vi "_UpdateTargetResFile.vi"(8 "error in (no error)":errorcluster, 10 "Polarity":enum32{"Positive", "Negative"}(radio), 11 "Path":path=path "C:/Users/Public/Molana/Instrument/Configuration/Current setting/Calibration/targetResolution.res") -> (0 "error out":errorcluster)   [LabVIEW 2015]
uses:
  Type/_Log Command.ctl
  Type/_RT Command.ctl
  Configuration/_Global Configuration.vi
  <vilib>/xml/Load XML File.vi
  <vilib>/xml/Close Reference(Node).vi
  <vilib>/xml/NI_XML.lvlib
  <resource>/objmgr/DOMUserDefRef.rc
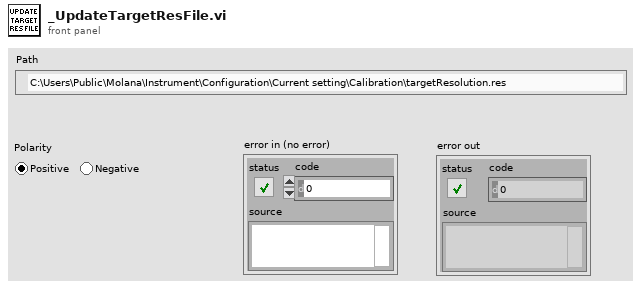
[diagram p1: front panel]
types:
  T1 = typedef "_Log Command.ctl" = enum16{"No Command", "Open", "Read", "Write", "Close", "Check Size"}
  T2 = typedef "_RT Command.ctl" = enum16{"xml Start Run", "xml Start Actual Run", "xml Stop Run", "xml Runtime Update", "xml Get Status", "xml Get Table", "xml Set Table", "xml Get Configuration", "xml System Status", "xml Set LC Input Logic", "xml Get Data", "xml Get Info", "Start", "StartActualRun", "Stop", "Runtime Update", "Get Data", "Get Info", "Get Status", "Get Param", "Get Config", "Get Table", "Read ADC", "Set Oscillator", "Update Config", "Update Table", "Set All Pol", "Set Pol and DC", "Set Max Mass", "Toggle RP", "Toggle EL", "Set PIC", "Initialize Turbo", "Send Turbo Comm", "Close Turbo", "P1", "P2", "P3", "Send Serial", "Set LC Out", "Get LC In", "Read VAC", "Test Table", "Toggle Power", "Get Startup", "Set Startup", "Get ADC Table", "Set ADC Table", "Get Brief Status", "Get Detail Status", "Auxiliary Update", "Set CC Logics", "Set CC Input Logics", "Ignore Error", "invalid"}
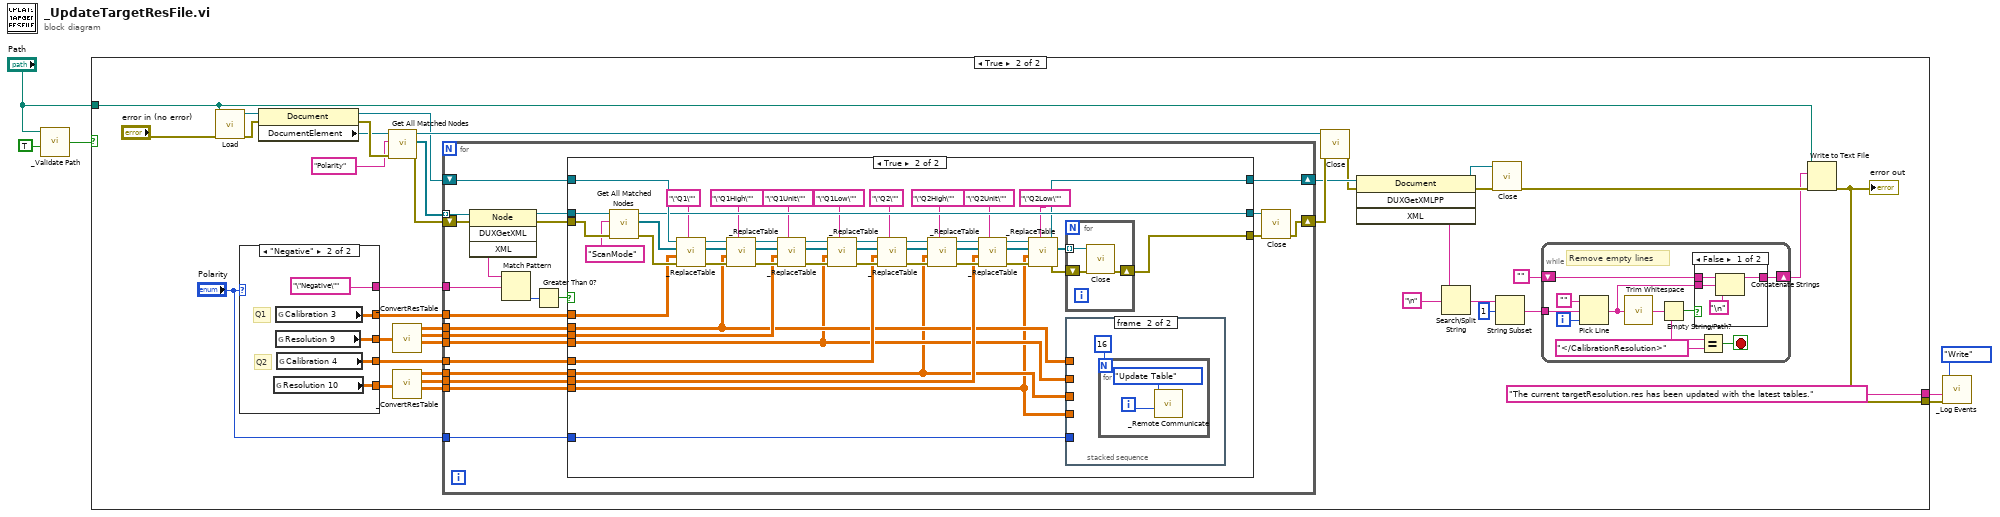
[diagram p0: block diagram]
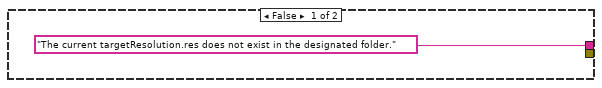
[diagram p2: hidden frame]
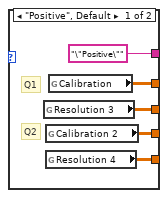
[diagram p4: hidden frame]
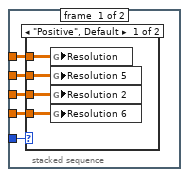
[diagram p6: hidden frame]
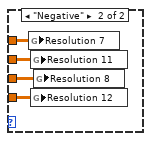
[diagram p7: hidden frame]
diagram:
  n1 = call "_Validate Path.vi"("Check Exist (F)"=TRUE, "path"="Path") -> ("Valid"=w4:bool)  [unwired: 2 in]
  n2 = case shown="True" w4 {
    tunnel: "Path" -> [_ w11]
    tunnel: ["The current targetResolution.res does not exist in the designated folder." ("initial string") "The current targetResolution.res has been updated with the latest tables." ("initial string")] -> w2
    tunnel: [_ w9] -> w1
    frame False {
    }
    frame True {
      n3 = call-poly <vilib>:"Load.vi"("path to XML document"=w11, "error in (no error)"="error in (no error)") -> ("DOM document out"=w45:refnum<k20>, "error out"=w44:errorcluster)  [unwired: 11 in, 1 out]
      n4 = case shown="\"Negative\"" "Polarity" {
        tunnel: ["\"Positive\"" "\"Negative\""] -> w38
        tunnel: [w64 w69] -> w32
        tunnel: [w63 w68] -> w34
        tunnel: [w62 w67] -> w31
        tunnel: [w61 w66] -> w33
        frame "Positive", Default {
          # "Q2"
          # "Q1"
          n5 = global read "_Global Configuration.vi" "Resolution 3"() -> (w63:dbl[][])
          n6 = global read "_Global Configuration.vi" "Calibration 2"() -> (w62:dbl[][])
          n7 = global read "_Global Configuration.vi" "Resolution 4"() -> (w61:dbl[][])
          n8 = global read "_Global Configuration.vi" "Calibration"() -> (w64:dbl[][])
        }
        frame "Negative" {
          # "Q2"
          # "Q1"
          n9 = global read "_Global Configuration.vi" "Resolution 10"() -> (w66:dbl[][])
          n10 = global read "_Global Configuration.vi" "Calibration 3"() -> (w69:dbl[][])
          n11 = global read "_Global Configuration.vi" "Resolution 9"() -> (w68:dbl[][])
          n12 = global read "_Global Configuration.vi" "Calibration 4"() -> (w67:dbl[][])
        }
      }
      n13 = property on="Property Node" class="Document"(reference=w45, error in=w44) -> (reference out=w35:refnum<k20>, error out=w43:errorcluster, "DocumentElement"=w42:refnum<k20>)
      n14 = call <vilib>:"Get All Matched Nodes.vi"("error in (no error)"=w43, "XPath expression"="Polarity", "node in"=w42) -> ("error out"=w40:errorcluster, "node result array"=w39:refnum<k20>[], "node out"=w36:refnum<k20>)  [unwired: 6 in]
      n15 = call "_ConvertResTable.vi"("ResTable"=w34) -> ("HiResTable"=w30:dbl[][], "MidResTable"=w29:dbl[][], "LowResTable"=w28:dbl[][])  [unwired: 1 in]
      n16 = call "_ConvertResTable.vi"("ResTable"=w33) -> ("HiResTable"=w27:dbl[][], "MidResTable"=w26:dbl[][], "LowResTable"=w25:dbl[][])  [unwired: 1 in]
      n17 = for {
        tunnel: w39 -> [w91] mode=indexing
        tunnel: w38 -> [w88]
        shift-right: [w86] -> w37
        shift-left: w40 -> [w92]
        shift-right: [w80] -> w24
        shift-left: w35 -> [w82]
        tunnel: w32 -> [w79]
        tunnel: w31 -> [w75]
        tunnel: w30 -> [w78]
        tunnel: w29 -> [w77]
        tunnel: w28 -> [w76]
        tunnel: w27 -> [w74]
        tunnel: w26 -> [w73]
        tunnel: w25 -> [w72]
        tunnel: "Polarity" -> [w71]
        n18 = invoke class="Node" method="DUXGetXML"(reference=w91, error in=w92) -> (reference out=w83:refnum<k20>, error out=w85:errorcluster, "XML"=w89:string)  [unwired: 2 in, 1 out]
        n19 = Match Pattern(string=w89, regular expression=w88) -> (offset past match=w90:i32)  [unwired: 1 in, 3 out]
        n20 = Greater Than 0?(x=w90) -> (x > 0?=w87:bool)
        n21 = case shown="True" w87 {
          tunnel: w85 -> [w95 w143]
          tunnel: [w95 w101] -> w84
          tunnel: w83 -> [w94 w144]
          tunnel: [w94 w139] -> w81
          tunnel: w82 -> [w93 w140]
          tunnel: [w93 w121] -> w80
          tunnel: w79 -> [_ w138]
          tunnel: w78 -> [_ w99]
          tunnel: w77 -> [_ w113]
          tunnel: w76 -> [_ w98]
          tunnel: w75 -> [_ w112]
          tunnel: w74 -> [_ w97]
          tunnel: w73 -> [_ w111]
          tunnel: w72 -> [_ w96]
          tunnel: w71 -> [_ w100]
          frame False {
          }
          frame True {
            n22 = call <vilib>:"Get All Matched Nodes.vi"("error in (no error)"=w143, "XPath expression"="ScanMode", "node in"=w144) -> ("error out"=w141:errorcluster, "node result array"=w114:refnum<k20>[], "node out"=w139:refnum<k20>)  [unwired: 6 in]
            n23 = call "_ReplaceTable.vi"("TableName"="\"Q1\"", "error in (no error)"=w141, "Table"=w138, "ScanModeRefArray"=w114, "DOM Document"=w140) -> ("error out"=w128:errorcluster, "ScanModeRefArrayOut"=w110:refnum<k20>[], "DOM DocumentOut"=w129:refnum<k20>)  [unwired: 1 in]
            n24 = call "_ReplaceTable.vi"("TableName"="\"Q1High\"", "error in (no error)"=w128, "Table"=w99, "ScanModeRefArray"=w110, "DOM Document"=w129) -> ("error out"=w127:errorcluster, "ScanModeRefArrayOut"=w109:refnum<k20>[], "DOM DocumentOut"=w120:refnum<k20>)  [unwired: 1 in]
            n25 = call "_ReplaceTable.vi"("TableName"="\"Q1Unit\"", "error in (no error)"=w127, "Table"=w113, "ScanModeRefArray"=w109, "DOM Document"=w120) -> ("error out"=w126:errorcluster, "ScanModeRefArrayOut"=w108:refnum<k20>[], "DOM DocumentOut"=w119:refnum<k20>)  [unwired: 1 in]
            n26 = call "_ReplaceTable.vi"("TableName"="\"Q1Low\"", "error in (no error)"=w126, "Table"=w98, "ScanModeRefArray"=w108, "DOM Document"=w119) -> ("error out"=w125:errorcluster, "ScanModeRefArrayOut"=w107:refnum<k20>[], "DOM DocumentOut"=w118:refnum<k20>)  [unwired: 1 in]
            n27 = call "_ReplaceTable.vi"("TableName"="\"Q2\"", "error in (no error)"=w125, "Table"=w112, "ScanModeRefArray"=w107, "DOM Document"=w118) -> ("error out"=w124:errorcluster, "ScanModeRefArrayOut"=w106:refnum<k20>[], "DOM DocumentOut"=w117:refnum<k20>)  [unwired: 1 in]
            n28 = call "_ReplaceTable.vi"("TableName"="\"Q2High\"", "error in (no error)"=w124, "Table"=w97, "ScanModeRefArray"=w106, "DOM Document"=w117) -> ("error out"=w123:errorcluster, "ScanModeRefArrayOut"=w105:refnum<k20>[], "DOM DocumentOut"=w116:refnum<k20>)  [unwired: 1 in]
            n29 = call "_ReplaceTable.vi"("TableName"="\"Q2Unit\"", "error in (no error)"=w123, "Table"=w111, "ScanModeRefArray"=w105, "DOM Document"=w116) -> ("error out"=w122:errorcluster, "ScanModeRefArrayOut"=w104:refnum<k20>[], "DOM DocumentOut"=w115:refnum<k20>)  [unwired: 1 in]
            n30 = call "_ReplaceTable.vi"("TableName"="\"Q2Low\"", "error in (no error)"=w122, "Table"=w96, "ScanModeRefArray"=w104, "DOM Document"=w115) -> ("error out"=w103:errorcluster, "ScanModeRefArrayOut"=w102:refnum<k20>[], "DOM DocumentOut"=w121:refnum<k20>)  [unwired: 1 in]
            n31 = for {
              tunnel: w102 -> [w163] mode=indexing
              shift-right: [w161] -> w101
              shift-left: w103 -> [w162]
              n32 = call-poly <vilib>:"Close.vi"("error in (no error)"=w162, "node"=w163) -> ("error out"=w161:errorcluster)  [unwired: 7 in]
            }
            n33 = stacked-sequence {
              tunnel: w100 -> [w149 _]
              tunnel: w99 -> [w148 _]
              tunnel: w98 -> [w147 _]
              tunnel: w97 -> [w146 _]
              tunnel: w96 -> [w145 _]
              frame #0 {
                n34 = case shown="\"Positive\", Default" w149 {
                  tunnel: w148 -> [w153 w157]
                  tunnel: w147 -> [w152 w156]
                  tunnel: w146 -> [w151 w155]
                  tunnel: w145 -> [w150 w154]
                  frame "Positive", Default {
                    n35 = global write "_Global Configuration.vi" "Resolution"(w153) -> ()
                    n36 = global write "_Global Configuration.vi" "Resolution 5"(w152) -> ()
                    n37 = global write "_Global Configuration.vi" "Resolution 2"(w151) -> ()
                    n38 = global write "_Global Configuration.vi" "Resolution 6"(w150) -> ()
                  }
                  frame "Negative" {
                    n39 = global write "_Global Configuration.vi" "Resolution 7"(w157) -> ()
                    n40 = global write "_Global Configuration.vi" "Resolution 11"(w156) -> ()
                    n41 = global write "_Global Configuration.vi" "Resolution 12"(w154) -> ()
                    n42 = global write "_Global Configuration.vi" "Resolution 8"(w155) -> ()
                  }
                }
              }
              frame #1 {
                n43 = for {
                  N: 16 -> [_]
                  i -> [w159]
                  n44 = call "_Remote Communicate.vi"("DC Param"=w159, "Command"=_RT_Command."Update Table") -> ()  [unwired: 4 in, 4 out]
                }
              }
            }
          }
        }
        n45 = call-poly <vilib>:"Close.vi"("error in (no error)"=w84, "node"=w81) -> ("error out"=w86:errorcluster)  [unwired: 7 in]
      }
      n46 = call-poly <vilib>:"Close.vi"("error in (no error)"=w37, "node"=w36) -> ("error out"=w23:errorcluster)  [unwired: 7 in]
      n47 = invoke class="Document" method="DUXGetXMLPP"(reference=w24, error in=w23) -> (reference out=w21:refnum<k20>, error out=w22:errorcluster, "XML"=w18:string)  [unwired: 2 in, 1 out]
      n48 = Search/Split String(string=w18, search string/char (-)="\n") -> (match + rest of string=w15:string)  [unwired: 1 in, 2 out]
      n49 = call-poly <vilib>:"Close.vi"("error in (no error)"=w22, "node"=w21) -> ("error out"=w16:errorcluster)  [unwired: 7 in]
      n50 = String Subset(string=w15, offset (0)=1) -> (substring=w14:string)  [unwired: 1 in]
      n51 = while {
        tunnel: w14 -> [w55]
        shift-right: [w51] -> w13
        shift-left: "" -> [w52]
        i -> [w54]
        stop <- w48 stop-if-true
        # "Remove empty lines"
        n52 = Pick Line(string ("")="", multi-line string=w55, line index=w54) -> (output string=w49:string)
        n53 = call <vilib>:"Trim Whitespace.vi"("string"=w49) -> ("trimmed string"=w47:string)  [unwired: 1 in]
        n54 = Empty String/Path?(string/path=w47) -> (empty?=w53:bool)
        n55 = case shown="False" w53 {
          tunnel: w52 -> [w59 w60]
          tunnel: [w57 w60] -> w51
          tunnel: w49 -> [w58 _]
          frame False {
            n56 = Concatenate Strings(w59, w58, "\n") -> (w57:string)
          }
          frame True {
          }
        }
        n57 = Equal?(x=w47, y="</CalibrationResolution>") -> (x = y?=w48:bool)
      }
      n58 = Write to Text File(file (use dialog)=w11, text=w13, error in=w16) -> (error out=w9:errorcluster)  [unwired: 1 in, 2 out]
      "error out" <- w9
    }
  }
  n59 = call "_Log Events.vi"("error in (no error)"=w1, "Event"=w2, "Log Command"=_Log_Command."Write") -> ()  [unwired: 5 in, 2 out]
